vi "Commit Transaction.vi"(8 "error in (no error)":errorcluster, 11 "Module ID":i32=-1) -> (0 "error out":errorcluster, 1 "timed out?":bool, 2 "Reply Payload":T1)   [LabVIEW 2014, in "DB_CONNECTOR.lvlib"]
doc: "Commit a transaction. Either all SQL-commands get commited or, in case of an error, all get rejected.\n_____\nCreated using Delacor QMH Event Scripter 4.0.0.68.\n\n<b>Note:</b> This VI was modified by the <b>Validate DQMH Module</b> tool to return an error if the reply times out."
uses:
  DB_CONNECTOR.lvlib
  Commit Transaction (Reply Payload)--cluster.ctl
  Commit Transaction Argument--cluster.ctl
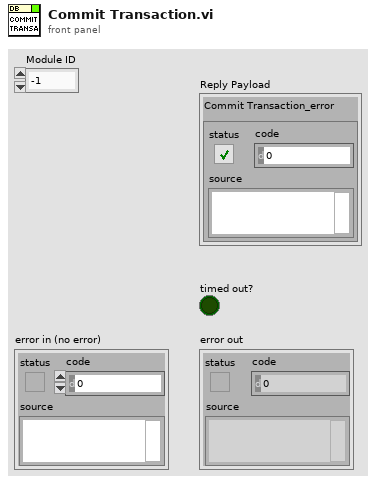
[diagram p1: front panel]
types:
  T1 = typedef "DB_CONNECTOR.lvlib/Commit Transaction (Reply Payload)--cluster.ctl" = cluster{"Commit Transaction_error":errorcluster}
  T2 = typedef "DB_CONNECTOR.lvlib/Commit Transaction Argument--cluster.ctl" = cluster{"Module ID":i32, "Wait Notifier":refnum<notifier>}
  T3 = typedef "DB_CONNECTOR.lvlib/Request Events--cluster.ctl" = cluster{"Stop Module":refnum<user-event>, "Show Panel":refnum<user-event>, "Hide Panel":refnum<user-event>, "Show Diagram":refnum<user-event>, "Get Module Execution Status":refnum<user-event>, "Configure":refnum<user-event>, "Connect":refnum<user-event>, "Query":refnum<user-event>, "Close Connection":refnum<user-event>, "Start Transaction":refnum<user-event>, "Commit Transaction":refnum<user-event>, "Fast Query":refnum<user-event>, "Get DB-Type":refnum<user-event>}
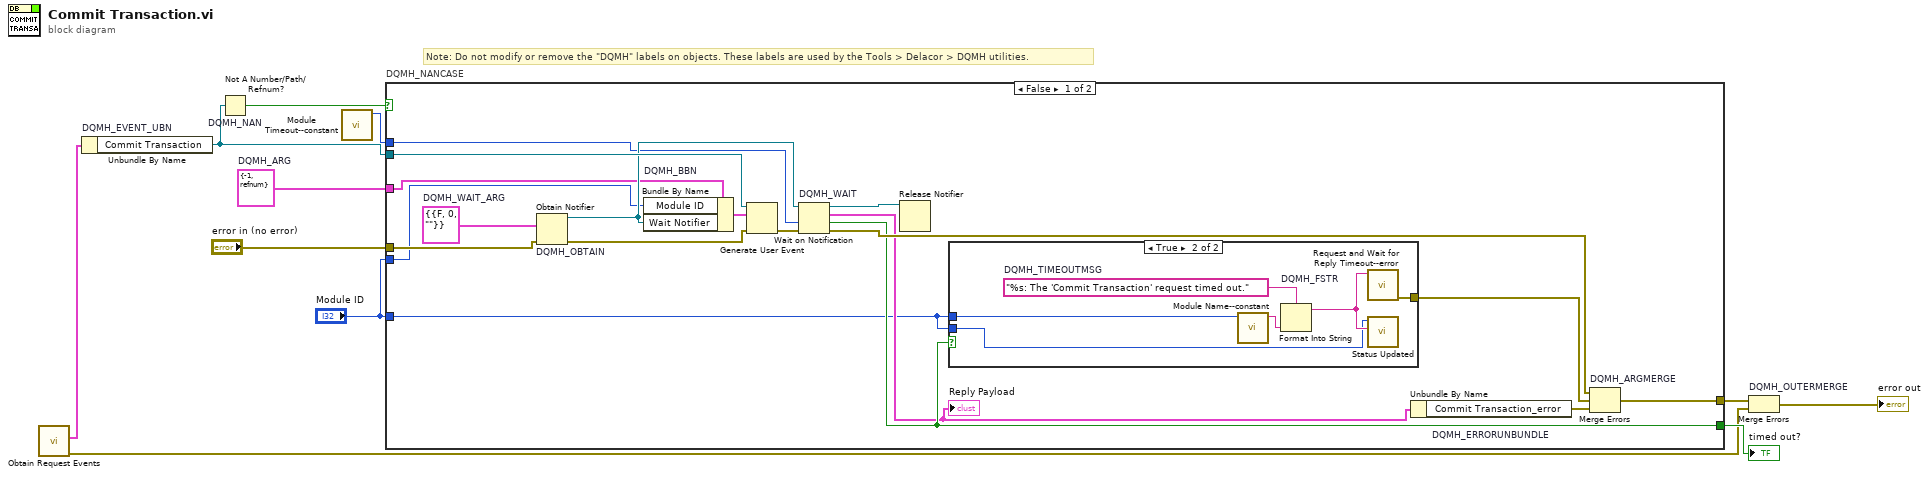
[diagram p0: block diagram]
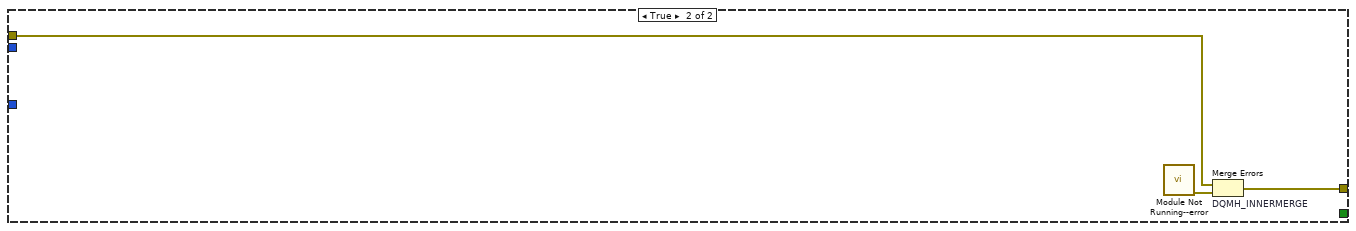
[diagram p3: hidden frame]
diagram:
  w5 = T2 {"Module ID"=-1, "Wait Notifier"=refnum}  # DQMH_ARG
  # "Note: Do not modify or remove the \"DQMH\" labels on objects. These labels are used by the Tools > Delacor > DQMH utilities."
  n1 = call "Obtain Request Events.vi"() -> ("error out"=w2:errorcluster, "DB_CONNECTOR Request Events"=w1:T3)  [unwired: 10 in]
  n2 = Unbundle By Name "DQMH_EVENT_UBN"(w1) -> ("Commit Transaction"=w9:refnum<user-event>)
  n3 = Not A Number/Path/Refnum? "DQMH_NAN"(number/path/refnum=w9) -> (NaN/Path/Refnum?=w8:bool)
  n4 = call "Module Timeout--constant.vi"() -> ("Module Timeout"=w4:i32)  [unwired: 11 in]
  n5 = case "DQMH_NANCASE" shown="False" w8 {
    tunnel: "error in (no error)" -> [w29 w38]
    tunnel: w9 -> [w27 _]
    tunnel: [w20 w37] -> w6
    tunnel: [w21 _] -> w7
    tunnel: w5 -> [w16 _]
    tunnel: "Module ID" -> [w15 _]
    tunnel: w4 -> [w14 _]
    tunnel: "Module ID" -> [w13 _]
    frame False {
      w25 = T1 {"Commit Transaction_error"={"status"=FALSE, "code"=0, "source"=""}}  # DQMH_WAIT_ARG
      n6 = Obtain Notifier "DQMH_OBTAIN"(notification data type=w25, error in (no error)=w29) -> (notifier out=w23:refnum<notifier>, error out=w26:errorcluster)  [unwired: 2 in, 1 out]
      n7 = Bundle By Name "DQMH_BBN"(cluster=w16, "Module ID"=w15, "Wait Notifier"=w23) -> (w17:T2)
      n8 = Generate User Event(user event=w27, event data cluster=w17, error in=w26) -> (error out=w28:errorcluster)  [unwired: 1 in, 1 out]
      n9 = Wait on Notification "DQMH_WAIT"(notifier=w23, timeout in ms (-1)=w14, error in (no error)=w28) -> (notifier out=w22:refnum<notifier>, notification=w18:T1, timed out?=w21:bool, error out=w24:errorcluster)  [unwired: 1 in]
      "Reply Payload" <- w18
      n10 = Release Notifier(notifier=w22) -> ()  [unwired: 2 in, 3 out]
      n11 = case shown="True" w21 {
        tunnel: w13 -> [_ w32]
        tunnel: w13 -> [_ w31]
        tunnel: [_ w30] -> w12
        frame False {
        }
        frame True {
          w35 = "%s: The 'Commit Transaction' request timed out."  # DQMH_TIMEOUTMSG
          n12 = call "Module Name--constant.vi"("Module ID"=w31) -> ("Module Name"=w34:string)  [unwired: 10 in]
          n13 = Format Into String "DQMH_FSTR"(format string=w35, w34) -> (resulting string=w33:string)  [unwired: 2 in, 1 out]
          n14 = call "Request and Wait for Reply Timeout--error.vi"("Error Message"=w33) -> ("error out"=w30:errorcluster)  [unwired: 10 in]
          n15 = call "Status Updated.vi"("Status"=w33, "Module ID"=w32) -> ()  [unwired: 9 in, 1 out]
        }
      }
      n16 = Unbundle By Name "DQMH_ERRORUNBUNDLE"(w18) -> ("Commit Transaction_error"=w19:errorcluster)
      n17 = Merge Errors "DQMH_ARGMERGE"(w24, w12, w19) -> (w20:errorcluster)
    }
    frame True {
      n18 = call "Module Not Running--error.vi"() -> ("error out"=w36:errorcluster)  [unwired: 11 in]
      n19 = Merge Errors "DQMH_INNERMERGE"(w38, w36) -> (w37:errorcluster)
    }
  }
  "timed out?" <- w7
  n20 = Merge Errors "DQMH_OUTERMERGE"(w6, w2) -> (→"error out":errorcluster)
